vi "Global Temperature.vi"(11 "Temp In":dbl[](array[numeric])) -> (2 "Std Out":dbl[](array[numeric]), 3 "Temp Out":dbl[](array[numeric]))   [LabVIEW 2018]
uses:
  <vilib>/Analysis/NI_AALBase.lvlib
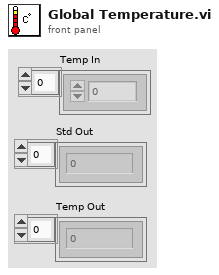
[diagram p1: front panel]
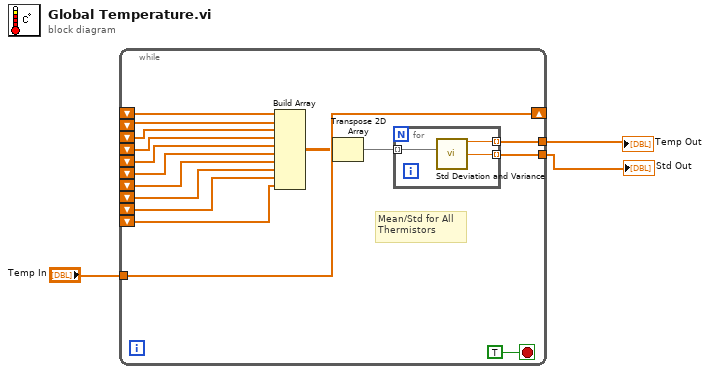
[diagram p0: block diagram]
diagram:
  n1 = while {
    tunnel: "Temp In" -> [w19]
    shift-right: [w19] -> _
    shift-left: _ -> [w15]
    shift-left: _ -> [w16]
    shift-left: _ -> [w17]
    shift-left: _ -> [w18]
    tunnel: [w14] -> w1
    tunnel: [w13] -> w2
    shift-left: _ -> [w9]
    shift-left: _ -> [w8]
    shift-left: _ -> [w7]
    shift-left: _ -> [w6]
    shift-left: _ -> [w5]
    shift-left: _ -> [w4]
    stop <- TRUE stop-if-true
    # "Mean/Std for All\nThermistors"
    n2 = Build Array(w18, w17, w16, w15, w9, w8, w7, w6, w5, w4) -> (w11:dbl[][])
    n3 = Transpose 2D Array(2D array=w11) -> (transposed array=w10:dbl[][])
    n4 = for {
      tunnel: w10 -> [w22] mode=indexing
      tunnel: [w21] -> w14 mode=indexing
      tunnel: [w20] -> w13 mode=indexing
      n5 = call <vilib>:"Std Deviation and Variance.vi"("X"=w22) -> ("mean"=w21:dbl, "standard deviation"=w20:dbl)  [unwired: 1 in, 1 out]
    }
  }
  "Temp Out" <- w1
  "Std Out" <- w2
